vi "Data_Delete.vi"(8 "error in (no error)":errorcluster, 11 "Ref In":T1 {"TS Parameter"."FCA" format="%01d"; "TS Parameter"."Target" min=1 max=100000; "TS Parameter"."PokaYoke" min=0 max=1}) -> (0 "error out":errorcluster)   [LabVIEW 2020]
uses:
  Controls/TD SQL.ctl
  <vilib>/addons/database/Connection.llb/Conn ObjectReference.ctl
  Controls/WIP_State.ctl
  Controls/TS_Parameter.ctl
  <vilib>/addons/database/NI_Database_API.lvlib
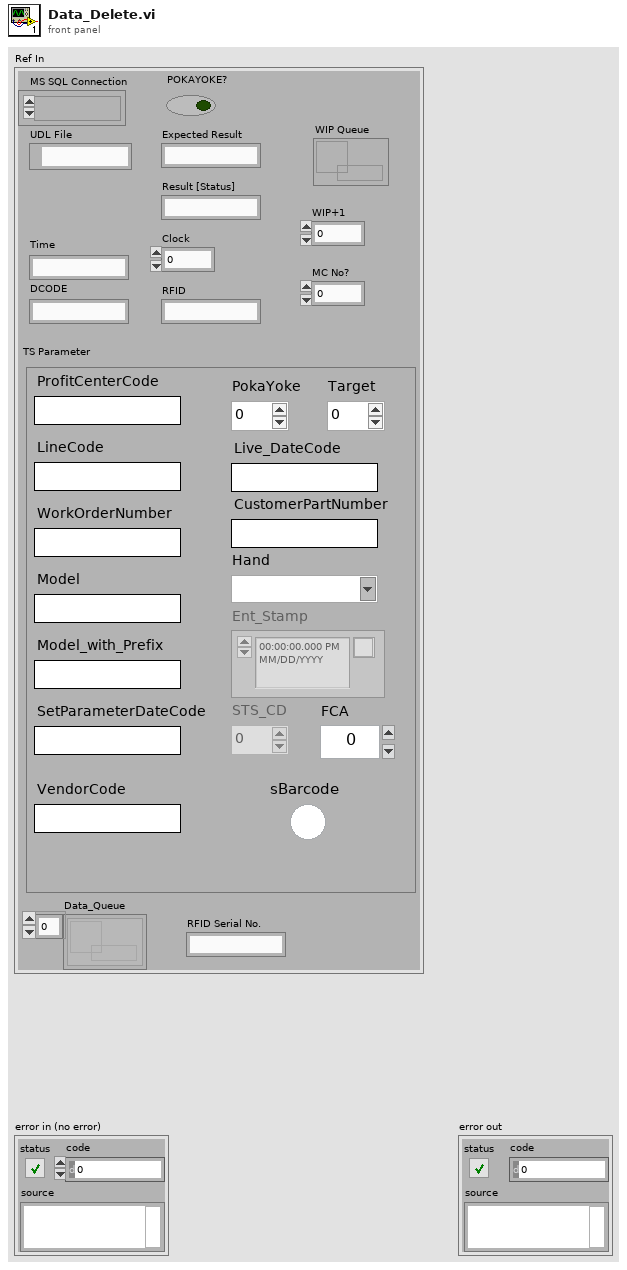
[diagram p1: front panel]
types:
  T1 = typedef "TD SQL.ctl" = cluster{"MS SQL Connection":T2, "UDL File":path, "Time":string, "DCODE":string, "WIP+1":i64, "MC No?":i32, "POKAYOKE?":bool, "Expected Result":string, "Result [Status]":string, "Clock":dbl, "RFID":string, "WIP Queue":refnum<queue>, "TS Parameter":T3, "Data_Queue":refnum<queue>[], "RFID Serial No.":string}
  T2 = typedef "NI_Database_API.lvlib/Conn ObjectReference.ctl" = refnum<k1>
  T3 = typedef "TS_Parameter.ctl" = cluster{"ProfitCenterCode":string, "LineCode":string, "WorkOrderNumber":string, "Model":string, "Model_with_Prefix":string, "VendorCode":string, "SetParameterDateCode":string, "PokaYoke":i32, "Target":i32, "Live_DateCode":string, "CustomerPartNumber":string, "Hand":string, "sBarcode":bool, "FCA":i32, "Ent_Stamp":timestamp, "STS_CD":dbl}
  T4 = enum32{"invalid app kind", "Development System", "Run Time System", "Student Edition", "Embedded LabVIEW", "Evaluation", "Custom"}
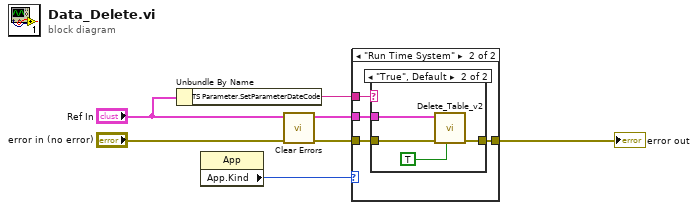
[diagram p0: block diagram]
diagram:
  n1 = Unbundle By Name("Ref In") -> ("TS Parameter.SetParameterDateCode"=w2:string)
  n2 = property class="App"() -> ("App.Kind"=w6:T4)  [unwired: 2 in, 2 out]
  n3 = call <vilib>:"Clear Errors.vi"("error in (no error)"="error in (no error)") -> ("error out"=w1:errorcluster)  [unwired: 5 in, 1 out]
  n4 = case shown="\"Run Time System\"" w6 {
    tunnel: "Ref In" -> [_ w10]
    tunnel: w1 -> [_ w9]
    tunnel: [_ w8] -> w5
    tunnel: w2 -> [_ w7]
    frame "invalid app kind", Default {
    }
    frame "Run Time System" {
      n5 = case shown="\"True\", Default" w7 {
        tunnel: w10 -> [_ w15]
        tunnel: w9 -> [w11 w14]
        tunnel: [w11 w12] -> w8
        frame "PKYK" {
        }
        frame "True", Default {
          n6 = call "Delete_Table_v2.vi"("Auto?"=TRUE, "error in (no error)"=w14, "Ref In"=w15) -> ("error out"=w12:errorcluster)  [unwired: 8 in]
        }
      }
    }
  }
  "error out" <- w5
